vi "temperature_logger_device.vi"(11 "Time Stamp":timestamp) -> (1 "Numeric":dbl, 2 "time string":string, 3 "date string":string)   [LabVIEW 2017]
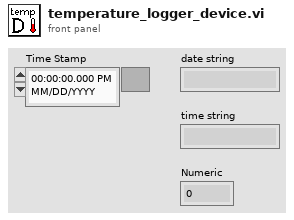
[diagram p1: front panel]
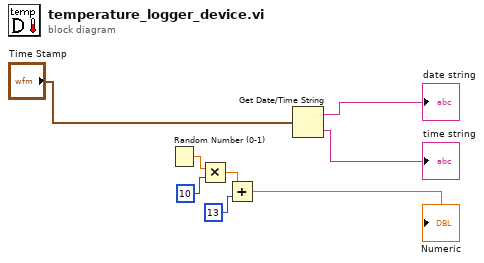
[diagram p0: block diagram]
diagram:
  n1 = Random Number (0-1)() -> (number: 0 to 1=w6:dbl)
  n2 = Multiply(x=w6, y=10) -> (x*y=w5:dbl)
  n3 = Add(x=w5, y=13) -> (x+y=→"Numeric":dbl)
  n4 = Get Date/Time String(seconds (now)="Time Stamp") -> (date string=→"date string":string, time string=→"time string":string)  [unwired: 2 in]
